vi "ini Ctrl_1D Var.vi"(5 "데이터타입":enum16{"I16", "U32"}(ring), 7 "Select":enum16{"Save", "Load"}(ring), 8 "에러 입력":errorcluster caption="에러 입력(에러 없음)", 9 "값":variant, 10 "키":string[](array[string]), 11 "섹션":string[](array[string])) -> (0 "에러 출력":errorcluster, 1 "값":string[](array[string]), 2 "경로 출력":path)   [LabVIEW 2020]
uses:
  Controls/Cmd_File path.ctl
  Controls/Cmd_File Type.ctl
  <vilib>/Utility/config.llb/Write Key (String).vi
  <vilib>/Utility/config.llb/Read Key (String).vi
  <vilib>/Utility/config.llb/NI_LVConfig.lvlib
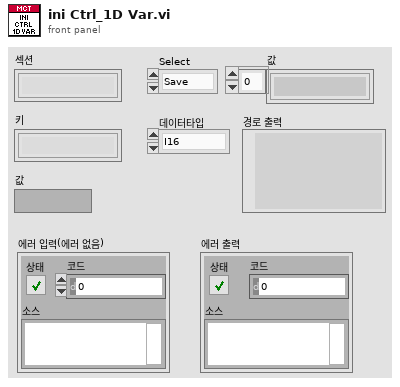
[diagram p1: front panel]
types:
  T1 = typedef "Cmd_File Type.ctl" = enum16{"엑셀", "엑셀(2003)", "텍스트", "설정", "2진", "VI", "CSV", "LOG", "폴더"}
  T2 = typedef "Cmd_File path.ctl" = enum16{"에러로그", "데이터파일경로", "성적서원본", "지난성적서", "Data Files", "경로생성", "Updater", "Template", "설정파일경로", "FTP Upload", "Update 경로", "어플리케이션"}
  T3 = typedef "NI_LVConfig.lvlib/Config Data RefNum.ctl" = refnum<k1>
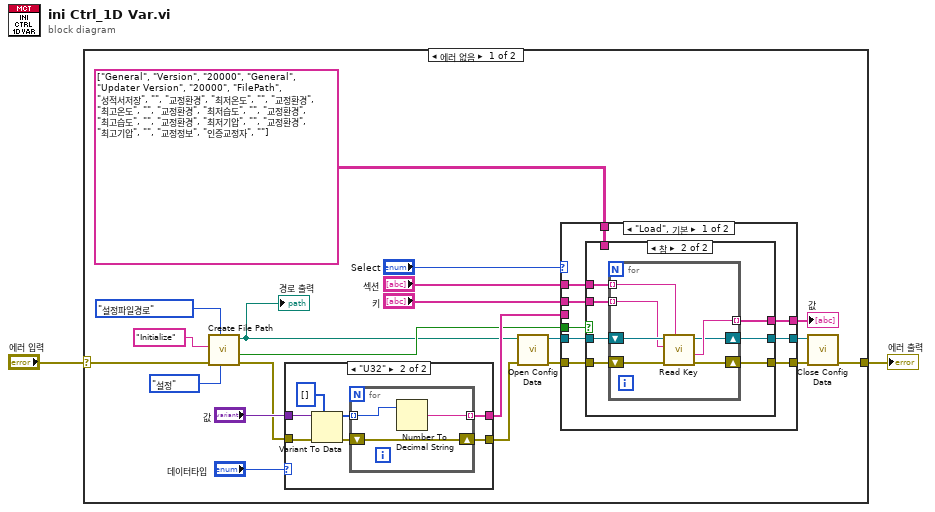
[diagram p0: block diagram]
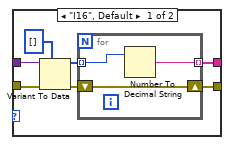
[diagram p2: hidden frame]
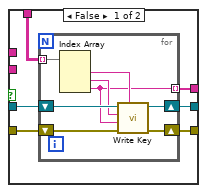
[diagram p3: hidden frame]
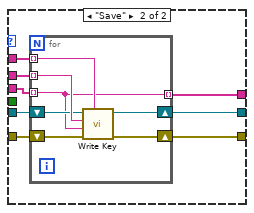
[diagram p4: hidden frame]
diagram:
  n1 = case shown="에러 없음" "에러 입력" {
    selector: "에러 입력" -> [w13 w96]
    tunnel: [w6 w96] -> w2
    frame No Error {
      n2 = call "Create File Path.vi"("파일타입"=Cmd_File_Type."설정", "항목"=Cmd_File_path."설정파일경로", "에러 입력"=w13, "문자열 in"="Initialize" ("파일명")) -> ("error out"=w14:errorcluster, "파일존재?"=w15:bool, "파일경로"=w11:path)  [unwired: 4 in, 1 out]
      "경로 출력" <- w11
      n3 = case shown="\"U32\"" "데이터타입" {
        tunnel: "값" -> [w29 w39]
        tunnel: w14 -> [w30 w40]
        tunnel: [w26 w36] -> w12
        tunnel: [w24 w34] -> w17
        frame "I16", Default {
          n4 = Variant To Data(error in=w30, type=i16[] [], Variant=w29) -> (data=w25:i16[], error out=w27:errorcluster)
          n5 = for {
            shift-right: [w32] -> w26
            shift-left: w27 -> [w32]
            tunnel: w25 -> [w33] mode=indexing
            tunnel: [w31] -> w24 mode=indexing
            n6 = Number To Decimal String(number=w33) -> (decimal integer string=w31:string)  [unwired: 1 in]
          }
        }
        frame "U32" {
          n7 = Variant To Data(error in=w40, type=u32[] [], Variant=w39) -> (data=w35:u32[], error out=w37:errorcluster)
          n8 = for {
            shift-right: [w42] -> w36
            shift-left: w37 -> [w42]
            tunnel: w35 -> [w43] mode=indexing
            tunnel: [w41] -> w34 mode=indexing
            n9 = Number To Decimal String(number=w43) -> (decimal integer string=w41:string)  [unwired: 1 in]
          }
        }
      }
      n10 = call <vilib>:"Open Config Data.vi"("error in (no error)"=w12, "configuration file path"=w11) -> ("error out"=w9:errorcluster, "refnum"=w10:T3)  [unwired: 7 in, 1 out]
      n11 = case shown="\"Load\", 기본" "Select" {
        tunnel: [w50 w82] -> w7
        tunnel: "키" -> [w47 w88]
        tunnel: "섹션" -> [w48 w87]
        tunnel: w9 -> [w52 w86]
        tunnel: w10 -> [w51 w85]
        tunnel: w15 -> [w49 _]
        tunnel: string[][] [["General", "Version", "20000"], ["General", "Updater Version", "20000"], ["FilePath", "성적서저장", ""], ["교정환경", "최저온도", ""], ["교정환경", "최고온도", ""], ["교정환경", "최저습도", ""], ["교정환경", "최고습도", ""], ["교정환경", "최저기압", ""], ["교정환경", "최고기압", ""], ["교정정보", "인증교정자", ""]] -> [w46 _]
        tunnel: w17 -> [_ w84]
        tunnel: [w45 w83] -> w8
        tunnel: [w44 w81] -> w5
        frame "Load", Default {
          n12 = case shown="참" w49 {
            tunnel: w52 -> [w56 w73]
            tunnel: w51 -> [w55 w72]
            tunnel: [w58 w69] -> w50
            tunnel: w48 -> [_ w71]
            tunnel: w47 -> [_ w70]
            tunnel: w46 -> [w57 _]
            tunnel: [w54 w68] -> w45
            tunnel: [w53 w67] -> w44
            frame False {
              n13 = for {
                shift-right: [w63] -> w58
                shift-left: w56 -> [w66]
                shift-right: [w64] -> w54
                shift-left: w55 -> [w65]
                tunnel: w57 -> [w62] mode=indexing
                tunnel: [w59] -> w53 mode=indexing
                n14 = Index Array(array=w62) -> (element #1=w61:string, element #2=w60:string, element #3=w59:string)  [unwired: 3 in]
                n15 = call-poly <vilib>:"Write Key.vi"("section"=w61, "error in (no error)"=w66, "value"=w59, "key"=w60, "refnum"=w65) -> ("error out"=w63:errorcluster, "refnum out"=w64:T3)  [unwired: 4 in, 1 out]
              }
            }
            frame True {
              n16 = for {
                tunnel: w71 -> [w78] mode=indexing
                tunnel: w70 -> [w77] mode=indexing
                tunnel: [w76] -> w67 mode=indexing
                shift-right: [w74] -> w69
                shift-left: w73 -> [w80]
                shift-right: [w75] -> w68
                shift-left: w72 -> [w79]
                n17 = call-poly <vilib>:"Read Key.vi"("section"=w78, "error in (no error)"=w80, "key"=w77, "refnum"=w79) -> ("error out"=w74:errorcluster, "value"=w76:string, "refnum out"=w75:T3)  [unwired: 4 in, 1 out]
              }
            }
          }
        }
        frame "Save" {
          n18 = for {
            tunnel: w88 -> [w93] mode=indexing
            tunnel: w87 -> [w92] mode=indexing
            tunnel: w84 -> [w89] mode=indexing
            shift-right: [w95] -> w83
            shift-left: w85 -> [w91]
            shift-right: [w94] -> w82
            shift-left: w86 -> [w90]
            tunnel: [w89] -> w81 mode=indexing
            n19 = call-poly <vilib>:"Write Key.vi"("section"=w92, "error in (no error)"=w90, "value"=w89, "key"=w93, "refnum"=w91) -> ("error out"=w94:errorcluster, "refnum out"=w95:T3)  [unwired: 4 in, 1 out]
          }
        }
      }
      "값" <- w5
      n20 = call <vilib>:"Close Config Data.vi"("error in (no error)"=w7, "refnum"=w8) -> ("error out"=w6:errorcluster)  [unwired: 8 in, 1 out]
    }
    frame Error {
    }
  }
  "에러 출력" <- w2
